vi "Read testActiveIsTrue.vi"(11 "TestMonitor in":refnum<class "TestMonitor.lvclass">) -> (2 "testActiveIsTrue":bool, 3 "TestMonitor out":refnum<class "TestMonitor.lvclass">)   [LabVIEW 2013, in "TestMonitor.lvclass"]
uses:
  TestMonitor.lvclass
  TestMonitor.lvclass/TestMonitor.ctl
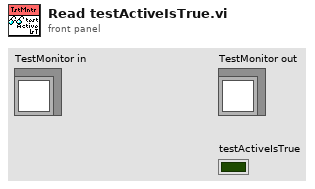
[diagram p1: front panel]
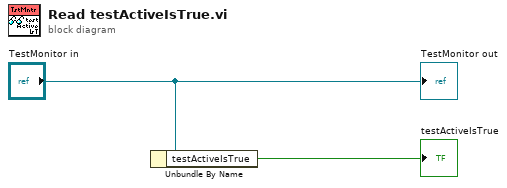
[diagram p0: block diagram]
diagram:
  n1 = Unbundle By Name("TestMonitor in") -> ("testActiveIsTrue"=→"testActiveIsTrue":bool)
  "TestMonitor out" <- "TestMonitor in"
